vi "Read Labels.vi"(8 "error in (no error)":errorcluster, 11 "Scanner in":refnum<class "Scanner.lvclass">) -> (0 "error out":errorcluster, 2 "Axis Label and Unit":T1[](array[typedef]), 3 "Scanner out":refnum<class "Scanner.lvclass">)   [LabVIEW 2017, in "Scanner.lvclass"]
uses:
  Scanner.lvclass
  Instruments/Utility Classes/Readable/Data Channel.ctl
  Instruments/Utility Classes/Readable/Data Point.ctl
  Instruments/Utility Classes/Readable/Time.ctl
  Instruments/Utility Classes/Readable/X.ctl
  Scanner.lvclass/Scanner.ctl
  Instruments/Utility Classes/Scannable/Scannable.lvclass
  Instruments/Utility Classes/Readable/Readable.lvclass
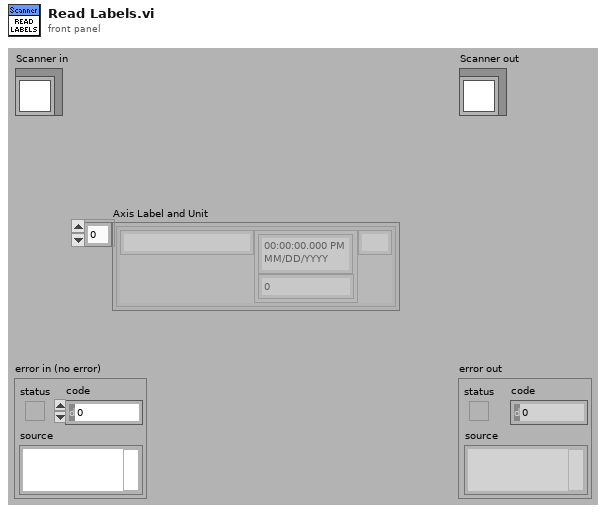
[diagram p1: front panel]
types:
  T1 = typedef "Readable.lvclass/Data Channel.ctl" = cluster{"Name":string, "Data Point":T2, "Unit":string}
  T2 = typedef "Readable.lvclass/Data Point.ctl" = cluster{"t":T3, "x":T4}
  T3 = typedef "Readable.lvclass/Time.ctl" = timestamp
  T4 = typedef "Readable.lvclass/X.ctl" = dbl
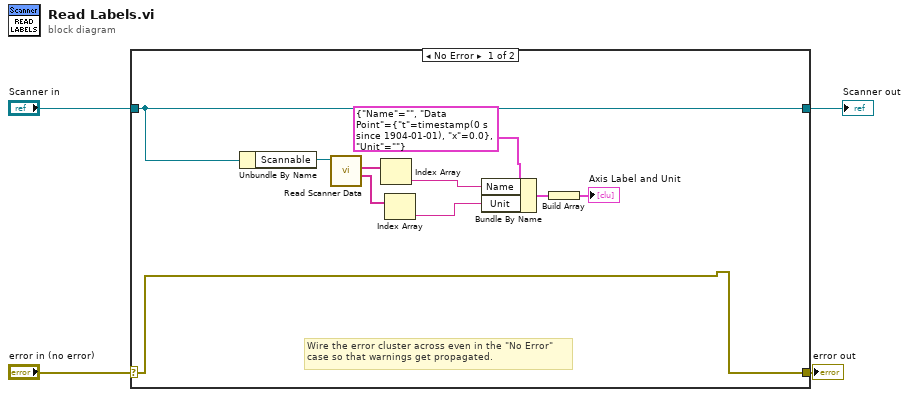
[diagram p0: block diagram]
diagram:
  n1 = case shown="No Error" "error in (no error)" {
    selector: "error in (no error)" -> [w14 w16]
    tunnel: [w14 w16] -> w3
    tunnel: [w12 w15] -> w1
    tunnel: "Scanner in" -> [w12 w15]
    frame No Error {
      # "Wire the error cluster across even in the \"No Error\"\ncase so that warnings get propagated."
      n2 = Unbundle By Name(w12) -> ("Scannable"=w13:refnum<class "Scannable.lvclass">)
      n3 = call-dynamic "Read Scanner Data.vi"("Scannable in"=w13) -> ("Channel Units"=w8:string[], "Channel Names"=w11:string[])  [unwired: 7 in, 2 out]
      n4 = Index Array(array=w11) -> (element=w10:string)  [unwired: 1 in]
      n5 = Index Array(array=w8) -> (element=w7:string)  [unwired: 1 in]
      n6 = Bundle By Name(cluster=T1 {"Name"="", "Data Point"={"t"=timestamp(0 s since 1904-01-01), "x"=0.0}, "Unit"=""} ("Add'l Data Channels"), "Name"=w10, "Unit"=w7) -> (w6:T1)
      n7 = Build Array(w6) -> (→"Axis Label and Unit":T1[])
    }
    frame Error {
    }
  }
  "error out" <- w3
  "Scanner out" <- w1
